vi "Read_Cals.vi"() -> ()   [LabVIEW 2019]
uses:
  <vilib>/Utility/file.llb/Read Delimited Spreadsheet (DBL).vi
  Globals/Flywheel_Globals.vi
panel:
  in  "default_LookupTable":dbl[][](array[numeric])=[[20.0, 5000.0], [70.0, 4800.0], [110.0, 4600.0], [130.0, 4600.0], [205.0, 4600.0], [260.0, 5000.0], [810.0, 5200.0]]
  out "all rows":dbl[][](array[numeric])
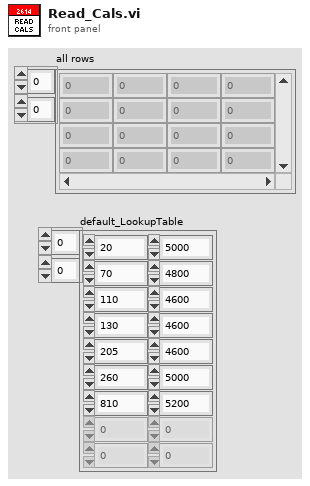
[diagram p1: front panel]
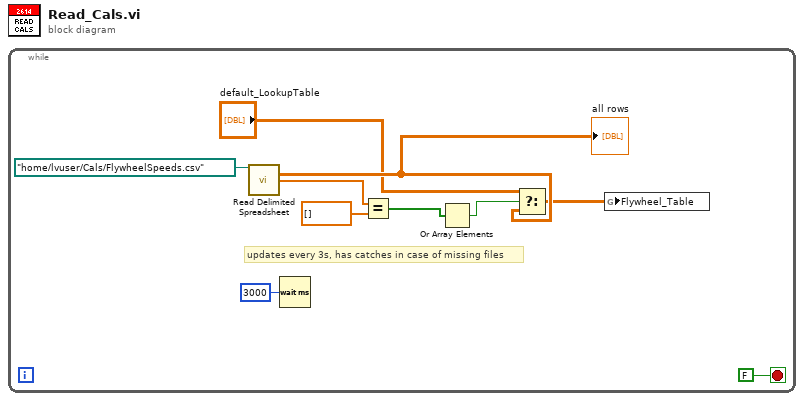
[diagram p0: block diagram]
diagram:
  n1 = while {
    stop <- FALSE stop-if-true
    # "updates every 3s, has catches in case of missing files"
    n2 = call-poly <vilib>:"Read Delimited Spreadsheet.vi"("file path (dialog if empty)"=path "/home/lvuser/Cals/FlywheelSpeeds.csv") -> ("all rows"=w5:dbl[][], "first row"=w7:dbl[])  [unwired: 9 in, 4 out]
    "all rows" <- w5
    n3 = Wait (ms)(milliseconds to wait=u32 3000) -> ()  [unwired: 1 out]
    n4 = Equal?(x=w7, y=dbl[] []) -> (x = y?=w3:bool[])
    n5 = Or Array Elements(Boolean array=w3) -> (logical OR=w2:bool)
    n6 = Select(t="default_LookupTable", s=w2, f=w5) -> (s? t:f=w1:dbl[][])
    n7 = global write "Flywheel_Globals.vi" "Flywheel_Table"(w1) -> ()
  }
